vi "Main.vi"(11 "Module Admin":refnum<class "Delacor_lib_QMH_Cloneable Module Admin.lvclass">) -> ()   [LabVIEW 2020, in "FGen.lvlib"]
doc: "This template is based off of the Queued Message Handler design pattern and the Queued Message Handler project template that ships with LabVIEW.\n\nThe main difference is that the queue is private to this module and communication between modules is performed via Broadcast and Request events.\n\nRequest events are wrapped in public API methods and are handled in the Event Handling Loop (EHL) of this VI. Any module can register for Broadcast events sent by this module. The EHL generates messages based on user interface actions.\n\nThe Message Handling Loop (MHL) processes messages generated by the EHL, or by other messages. The messages are string values, so new messages can be added easily to the Message Cases case structure in the MHL. Each message cluster can also provide an optional value for Message Data, which is a variant that can be converted to whatever message-specific data is required.\n_____\nBased on DQMH Project Template 6.0.0.91."
uses:
  FGen.lvlib
  <vilib>/Delacor/Delacor QMH/Libraries/Message Queue_class/Delacor_lib_QMH_Message Queue.lvclass
  Module Data--cluster.ctl
  <vilib>/Utility/miscctls.llb/LVPointTypeDef.ctl
  <vilib>/Utility/error.llb/Error Cluster From Error Code.vi
  <vilib>/ErrorRing/Error Ring.xnode
  <vilib>/Delacor/Delacor QMH/Libraries/Message Queue_class/Delacor_lib_QMH_Enqueue Message (Single).vi
  Stop Argument--cluster.ctl
  <vilib>/Delacor/Delacor QMH/Libraries/Cloneable Module Admin_class/Delacor_lib_QMH_Cloneable Module Admin.lvclass
  Set Signal Type Argument--cluster.ctl
  Clases/Generador/Generador.lvclass
  Set to Default Argument--cluster.ctl
  Generate Signal (Reply Payload)--cluster.ctl
  Generate Signal Argument--cluster.ctl
  Oscilloscope Lista Argument--cluster.ctl
panel:
  out "error out":errorcluster
  out "Status":string
  in  "Simulate EHL Error":bool
  in  "Simulate MHL Error":bool
  # "Other QMH Modules communicate with this Module via its Public API (wrappers for its Request Events).\n\nThis Module communicates with other Modules via its Broadcast Events.\nAny module that wants to get these messages, just registers for this module's Broadcast events."
  # "This template is for the Delacor Modified Queued Message Handler design pattern.\n\nSee the block diagram for more information on how to use this template."
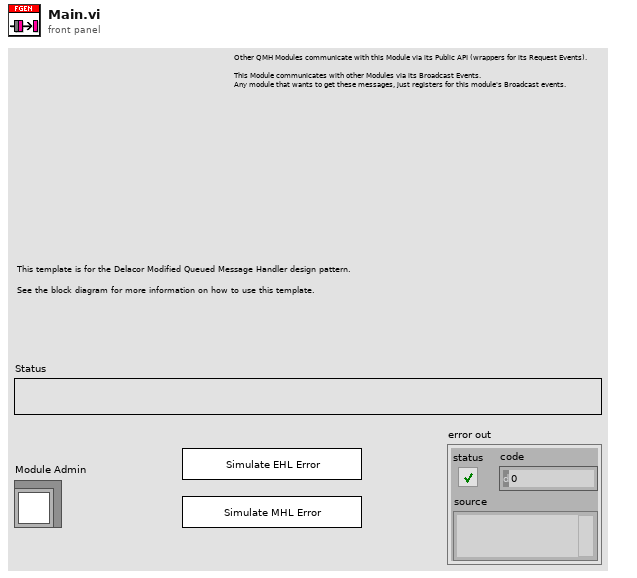
[diagram p1: front panel]
types:
  T1 = typedef "FGen.lvlib/Request Events--cluster.ctl" = cluster{"Stop Module":refnum<user-event>, "Show Panel":refnum<user-event>, "Hide Panel":refnum<user-event>, "Show Diagram":refnum<user-event>, "Get Module Execution Status":refnum<user-event>, "Set Signal Type":refnum<user-event>, "Set to Default":refnum<user-event>, "Generate Signal":refnum<user-event>}
  T2 = typedef "FGen.lvlib/Module Data--cluster.ctl" = cluster{"Status":string, "Generator":refnum<class "Generador.lvclass">}
  T3 = enum32{"invalid lock state", "Not Locked", "Locked (No Password)", "Password-protected"}
  T4 = typedef "FGen.lvlib/Stop Argument--cluster.ctl" = cluster{"Module ID":i32, "Origin":string, "Exit via Stop Module Req?":bool, "Wait for Module to stop?":bool}
  T5 = typedef "FGen.lvlib/Set Signal Type Argument--cluster.ctl" = cluster{"Module ID":i32, "signal type":enum16{"Sine Wave", "Triangle Wave", "Square Wave", "Sawtooth Wave"}}
  T6 = typedef "FGen.lvlib/Set to Default Argument--cluster.ctl" = cluster{"Module ID":i32, "Boolean":bool}
  T7 = typedef "FGen.lvlib/Generate Signal Argument--cluster.ctl" = cluster{"Module ID":i32, "Wait Notifier":refnum<notifier>, "wait for reply":bool}
  T8 = typedef "LVPointTypeDef.ctl" = cluster{"Horizontal":i16, "Vertical":i16}
  T9 = enum32{"Invalid", "Standard", "Closed", "Hidden", "Minimized", "Maximized"}
  T10 = typedef "FGen.lvlib/Generate Signal (Reply Payload)--cluster.ctl" = cluster{"signal out":waveform(dbl), "Generate Signal_error":errorcluster}
  T11 = typedef "FGen.lvlib/Oscilloscope Lista Argument--cluster.ctl" = cluster{"Module ID":i32, "Oscilloscopes Types":string[]}
  T12 = enum16{"Sine Wave", "Triangle Wave", "Square Wave", "Sawtooth Wave"}
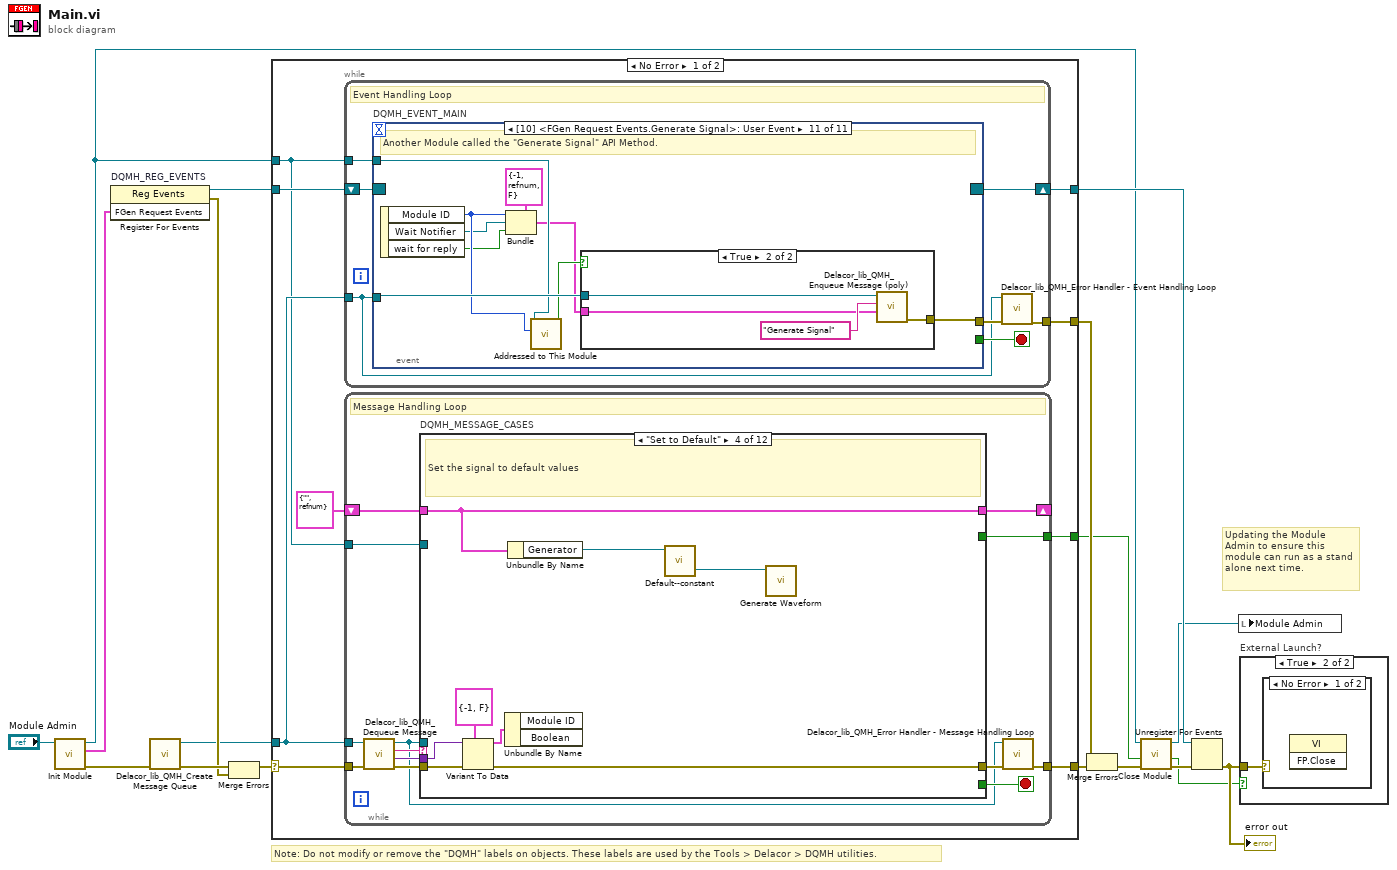
[diagram p0: block diagram]
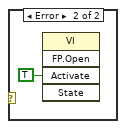
[diagram p3: hidden frame]
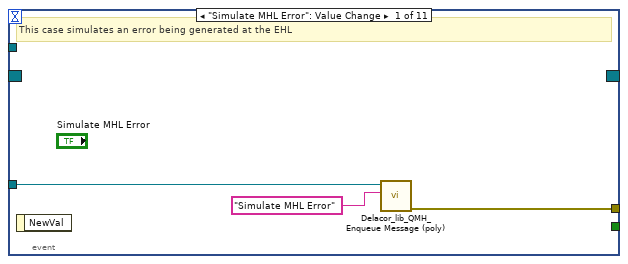
[diagram p4: hidden frame]
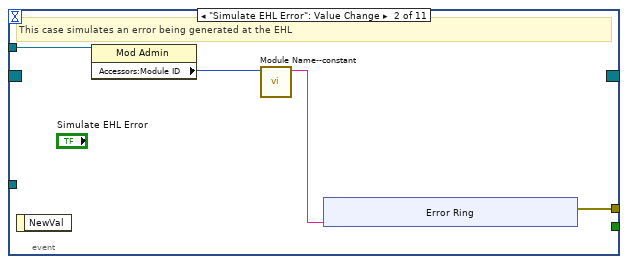
[diagram p5: hidden frame]
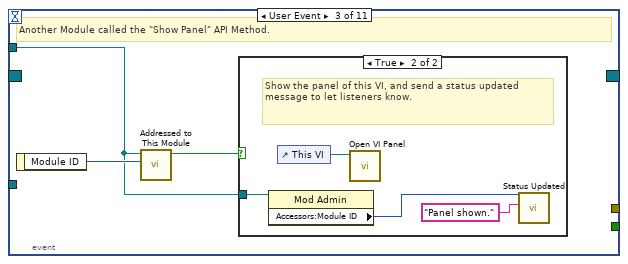
[diagram p6: hidden frame]
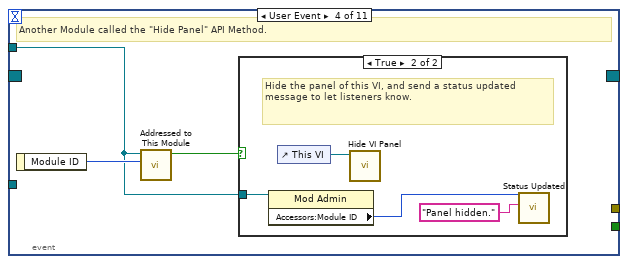
[diagram p8: hidden frame]
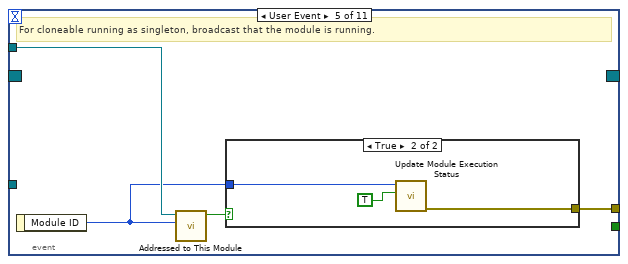
[diagram p10: hidden frame]
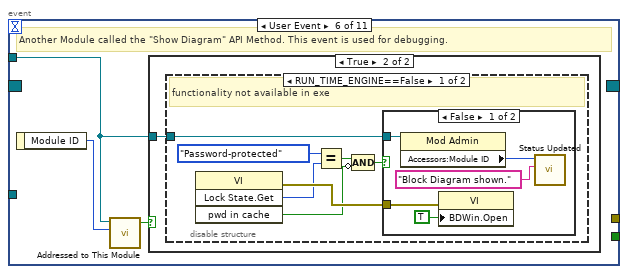
[diagram p12: hidden frame]
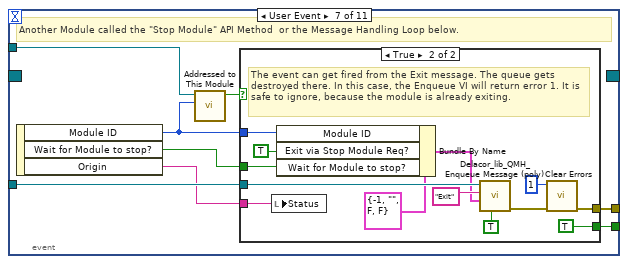
[diagram p16: hidden frame]
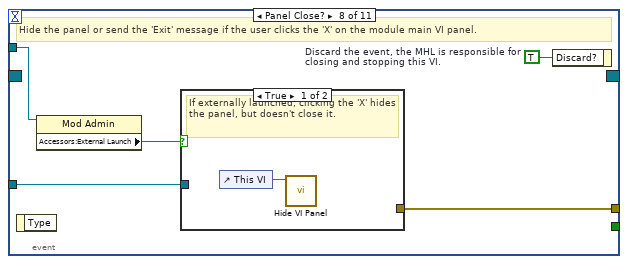
[diagram p18: hidden frame]
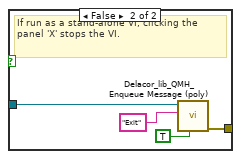
[diagram p19: hidden frame]
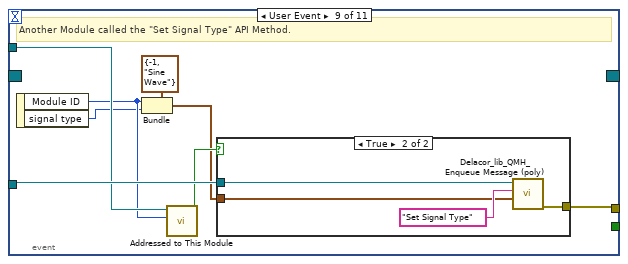
[diagram p20: hidden frame]
diagram:
  # "Note: Do not modify or remove the \"DQMH\" labels on objects. These labels are used by the Tools > Delacor > DQMH utilities."
  # "Updating the Module Admin to ensure this module can run as a stand alone next time."
  n1 = call "Init Module.vi"("Cloneable Module Admin in"="Module Admin") -> ("error out"=w15:errorcluster, "FGen Request Events"=w7:T1, "Cloneable Module Admin out"=w4:refnum<class "Delacor_lib_QMH_Cloneable Module Admin.lvclass">)  [unwired: 8 in]
  n2 = register-events "DQMH_REG_EVENTS"(w7) -> (reference out=w8:refnum<event-registration>, error out=w10:errorcluster)  [unwired: 2 in]
  n3 = call <vilib>:"Delacor_lib_QMH_Create Message Queue.vi"("error in"=w15) -> ("error out"=w12:errorcluster, "Message Queue"=w6:refnum<class "Delacor_lib_QMH_Message Queue.lvclass">)  [unwired: 9 in]
  n4 = Merge Errors(w12, w10) -> (w11:errorcluster)
  n5 = case shown="No Error" w11 {
    selector: w11 -> [w25 w300]
    tunnel: [w27 w299] -> w16
    tunnel: [w24 w307] -> w9
    tunnel: w8 -> [w22 w307]
    tunnel: w6 -> [w21 w298]
    tunnel: [w26 _] -> w17
    tunnel: w4 -> [w20 w303]
    tunnel: [w19 _] -> w2
    frame No Error {
      n6 = while {
        tunnel: w21 -> [w28]
        shift-right: [w31] -> w24
        shift-left: w22 -> [w32]
        tunnel: [w33] -> w26
        tunnel: w20 -> [w29]
        stop <- w30 stop-if-true
        # "Event Handling Loop"
        n7 = event "DQMH_EVENT_MAIN" shown="[10] <FGen Request Events.Generate Signal>: User Event" {
          selector: w32 -> [_ _ _ _ _ _ _ _ _ _ _]
          dyn-events: [_ _ _ _ _ _ _ _ _ _ _] -> w31
          timeout: _ -> [_ _ _ _ _ _ _ _ _ _ _]
          tunnel: [_ _ _ _ _ _ w89 _ _ _ _] -> w30
          tunnel: w28 -> [w36 _ _ _ _ _ w92 w108 w124 w136 w149]
          tunnel: [w37 w41 _ _ w66 _ w93 w111 w117 w129 w141] -> w34
          tunnel: w29 -> [_ w40 w49 w56 w64 w70 w91 w109 w122 w134 w147]
          event "Simulate MHL Error": Value Change {
            # "This case simulates an error being generated at the EHL"
            n8 = event-data() -> ()  [unwired: 1 in, 1 out]
            n9 = call-poly <vilib>:"Delacor_lib_QMH_Enqueue Message (poly).vi"("Message"="Simulate MHL Error", "Message Queue in"=w36) -> ("error out"=w37:errorcluster)  [unwired: 8 in, 1 out]
          }
          event "Simulate EHL Error": Value Change {
            # "This case simulates an error being generated at the EHL"
            n10 = event-data() -> ()  [unwired: 1 in, 1 out]
            n11 = property class="Mod Admin"(reference=w40) -> ("Accessors:Module ID"=w39:i32)  [unwired: 1 in, 2 out]
            n12 = call "Module Name--constant.vi"("Module ID"=w39) -> ("Module Name"=w38:string)  [unwired: 10 in]
            n13 = xnode "Error Ring"("parameter 0"=w38) -> ("error out"=w41:errorcluster)
          }
          event User Event {
            # "Another Module called the \"Show Panel\" API Method."
            n14 = event-data() -> ("Module ID"=w50:i32)  [unwired: 1 in]
            n15 = call "Addressed to This Module.vi"("Module ID from Argument"=w50, "Module Admin"=w49) -> ("Addressed to this instance?"=w51:bool)  [unwired: 8 in, 1 out]
            n16 = case shown="True" w51 {
              tunnel: w49 -> [_ w53]
              frame False {
              }
              frame True {
                # "Show the panel of this VI, and send a status updated message to let listeners know."
                n17 = property class="Mod Admin"(reference=w53) -> ("Accessors:Module ID"=w52:i32)  [unwired: 1 in, 2 out]
                n18 = control-ref of="This VI"() -> (w55:refnum<vi>)
                n19 = call "Open VI Panel.vi"("VI"=w55) -> ()  [unwired: 10 in, 1 out]
                n20 = call "Status Updated.vi"("Status"="Panel shown." ("format string"), "Module ID"=w52) -> ()  [unwired: 9 in, 1 out]
              }
            }
          }
          event User Event {
            # "Another Module called the \"Hide Panel\" API Method."
            n21 = event-data() -> ("Module ID"=w57:i32)  [unwired: 1 in]
            n22 = call "Addressed to This Module.vi"("Module ID from Argument"=w57, "Module Admin"=w56) -> ("Addressed to this instance?"=w58:bool)  [unwired: 8 in, 1 out]
            n23 = case shown="True" w58 {
              tunnel: w56 -> [_ w60]
              frame False {
              }
              frame True {
                # "Hide the panel of this VI, and send a status updated message to let listeners know."
                n24 = property class="Mod Admin"(reference=w60) -> ("Accessors:Module ID"=w59:i32)  [unwired: 1 in, 2 out]
                n25 = control-ref of="This VI"() -> (w62:refnum<vi>)
                n26 = call "Hide VI Panel.vi"("VI"=w62) -> ()  [unwired: 10 in, 1 out]
                n27 = call "Status Updated.vi"("Status"="Panel hidden." ("format string"), "Module ID"=w59) -> ()  [unwired: 9 in, 1 out]
              }
            }
          }
          event User Event {
            # "For cloneable running as singleton, broadcast that the module is running."
            n28 = event-data() -> ("Module ID"=w63:i32)  [unwired: 1 in]
            n29 = call "Addressed to This Module.vi"("Module ID from Argument"=w63, "Module Admin"=w64) -> ("Addressed to this instance?"=w65:bool)  [unwired: 8 in, 1 out]
            n30 = case shown="True" w65 {
              tunnel: [_ w69] -> w66
              tunnel: w63 -> [_ w68]
              frame False {
              }
              frame True {
                n31 = call "Update Module Execution Status.vi"("Running?"=TRUE, "Module ID"=w68) -> ("error out"=w69:errorcluster)  [unwired: 9 in]
              }
            }
          }
          event User Event {
            # "Another Module called the \"Show Diagram\" API Method. This event is used for debugging."
            n32 = event-data() -> ("Module ID"=w71:i32)  [unwired: 1 in]
            n33 = call "Addressed to This Module.vi"("Module ID from Argument"=w71, "Module Admin"=w70) -> ("Addressed to this instance?"=w72:bool)  [unwired: 8 in, 1 out]
            n34 = case shown="True" w72 {
              tunnel: w70 -> [_ w73]
              frame False {
              }
              frame True {
                n35 = disable-structure shown="RUN_TIME_ENGINE==False" {
                  disable-tunnel: w73 -> [w74 _]
                  frame condition #0 (active) {
                    # "functionality not available in exe"
                    n36 = invoke class="VI" method="Lock State.Get"() -> (error out=w80:errorcluster, "Get Lock State"=w79:T3, "pwd in cache"=w76:bool)  [unwired: 4 in, 1 out]
                    n37 = Equal?(x=T3."Password-protected", y=w79) -> (x = y?=w77:bool)
                    n38 = Compound Arithmetic op=AND(w77, invert w76) -> (w75:bool)
                    n39 = case shown="False" w75 {
                      tunnel: w80 -> [w85 _]
                      tunnel: w74 -> [w82 _]
                      frame False {
                        n40 = property class="Mod Admin"(reference=w82) -> ("Accessors:Module ID"=w81:i32)  [unwired: 1 in, 2 out]
                        n41 = property class="VI"(error in=w85, "BDWin.Open"=TRUE ("Block Diagram Window:Open")) -> ()  [unwired: 1 in, 2 out]
                        n42 = call "Status Updated.vi"("Status"="Block Diagram shown." ("format string"), "Module ID"=w81) -> ()  [unwired: 9 in, 1 out]
                      }
                      frame True {
                        # "Password-protected VI, and the password is not in the cache. Do not show the diagram."
                      }
                    }
                  }
                  frame condition #1 {
                  }
                }
              }
            }
          }
          event User Event {
            # "Another Module called the \"Stop Module\" API Method  or the Message Handling Loop below."
            n43 = event-data() -> ("Module ID"=w87:i32, "Wait for Module to stop?"=w88:bool, "Origin"=w86:string)  [unwired: 1 in]
            n44 = call "Addressed to This Module.vi"("Module ID from Argument"=w87, "Module Admin"=w91) -> ("Addressed to this instance?"=w90:bool)  [unwired: 8 in, 1 out]
            n45 = case shown="True" w90 {
              tunnel: [_ w105] -> w93
              tunnel: w92 -> [_ w101]
              tunnel: [_ TRUE] -> w89
              tunnel: w88 -> [_ w96]
              tunnel: w87 -> [_ w98]
              tunnel: w86 -> [_ w94]
              frame False {
              }
              frame True {
                # "The event can get fired from the Exit message. The queue gets destroyed there. In this case, the Enqueue VI will return error 1. It is safe to ignore, because the module is already exiting."
                n46 = local write "Status"(w94) -> ()
                n47 = Bundle By Name(cluster=T4 {"Module ID"=-1, "Origin"="", "Exit via Stop Module Req?"=FALSE, "Wait for Module to stop?"=FALSE} ("Stop Argument"), "Module ID"=w98, "Exit via Stop Module Req?"=TRUE, "Wait for Module to stop?"=w96) -> (w95:T4)
                n48 = call-poly <vilib>:"Delacor_lib_QMH_Enqueue Message (poly).vi"("Priority Message? (F)"=TRUE, "Message Data"=w95, "Message"="Exit", "Message Queue in"=w101) -> ("error out"=w106:errorcluster)  [unwired: 6 in, 1 out]
                n49 = call <vilib>:"Clear Errors.vi"("error in (no error)"=w106, "specific error code to clear (0: all)"=1) -> ("error out"=w105:errorcluster)  [unwired: 4 in, 1 out]
              }
            }
          }
          event Panel Close? {
            w110 = TRUE  # Discard the event, the MHL is responsible for closing and stopping this VI.
            # "Hide the panel or send the 'Exit' message if the user clicks the 'X' on the module main VI panel."
            n50 = event-data() -> ()  [unwired: 1 in, 1 out]
            n51 = property class="Mod Admin"(reference=w109) -> ("Accessors:External Launch"=w107:bool)  [unwired: 1 in, 2 out]
            n52 = case shown="True" w107 {
              tunnel: w108 -> [_ w115]
              tunnel: [_ w116] -> w111
              frame True {
                # "If externally launched, clicking the 'X' hides the panel, but doesn't close it."
                n53 = control-ref of="This VI"() -> (w112:refnum<vi>)
                n54 = call "Hide VI Panel.vi"("VI"=w112) -> ()  [unwired: 10 in, 1 out]
              }
              frame False {
                # "If run as a stand-alone VI, clicking the panel 'X' stops the VI."
                n55 = call-poly <vilib>:"Delacor_lib_QMH_Enqueue Message (poly).vi"("Priority Message? (F)"=TRUE, "Message"="Exit", "Message Queue in"=w115) -> ("error out"=w116:errorcluster)  [unwired: 7 in, 1 out]
              }
            }
            n56 = event-data("Discard?"=w110) -> ()  [unwired: 1 in, 1 out]
          }
          event User Event {
            # "Another Module called the \"Set Signal Type\" API Method."
            n57 = event-data() -> ("Module ID"=w119:i32, "signal type"=w118:T12)  [unwired: 1 in]
            n58 = Bundle(cluster=T5 {"Module ID"=-1, "signal type"=enum."Sine Wave"} ("Set Signal Type Argument"), "Module ID"=w119, "signal type"=w118) -> (w120:T5)
            n59 = call "Addressed to This Module.vi"("Module ID from Argument"=w119, "Module Admin"=w122) -> ("Addressed to this instance?"=w123:bool)  [unwired: 8 in, 1 out]
            n60 = case shown="True" w123 {
              tunnel: w124 -> [_ w128]
              tunnel: w120 -> [_ w126]
              tunnel: [_ w125] -> w117
              frame False {
              }
              frame True {
                n61 = call-poly <vilib>:"Delacor_lib_QMH_Enqueue Message (poly).vi"("Message Data"=w126, "Message"="Set Signal Type", "Message Queue in"=w128) -> ("error out"=w125:errorcluster)  [unwired: 7 in, 1 out]
              }
            }
          }
          event User Event {
            # "Another Module called the \"Set to Default\" API Method."
            n62 = event-data() -> ("Module ID"=w131:i32, "Boolean"=w130:bool)  [unwired: 1 in]
            n63 = Bundle(cluster=T6 {"Module ID"=-1, "Boolean"=FALSE} ("Set to Default Argument"), "Module ID"=w131, "Boolean"=w130) -> (w132:T6)
            n64 = call "Addressed to This Module.vi"("Module ID from Argument"=w131, "Module Admin"=w134) -> ("Addressed to this instance?"=w135:bool)  [unwired: 8 in, 1 out]
            n65 = case shown="True" w135 {
              tunnel: w136 -> [_ w140]
              tunnel: w132 -> [_ w138]
              tunnel: [_ w137] -> w129
              frame False {
              }
              frame True {
                n66 = call-poly <vilib>:"Delacor_lib_QMH_Enqueue Message (poly).vi"("Message Data"=w138, "Message"="Set to Default", "Message Queue in"=w140) -> ("error out"=w137:errorcluster)  [unwired: 7 in, 1 out]
              }
            }
          }
          event User Event {
            # "Another Module called the \"Generate Signal\" API Method."
            n67 = event-data() -> ("Module ID"=w144:i32, "Wait Notifier"=w143:refnum<notifier>, "wait for reply"=w142:bool)  [unwired: 1 in]
            n68 = Bundle(cluster=T7 {"Module ID"=-1, "Wait Notifier"=refnum, "wait for reply"=FALSE} ("Generate Signal Argument"), "Module ID"=w144, "Wait Notifier"=w143, "wait for reply"=w142) -> (w145:T7)
            n69 = call "Addressed to This Module.vi"("Module ID from Argument"=w144, "Module Admin"=w147) -> ("Addressed to this instance?"=w148:bool)  [unwired: 8 in, 1 out]
            n70 = case shown="True" w148 {
              tunnel: w149 -> [_ w153]
              tunnel: w145 -> [_ w151]
              tunnel: [_ w150] -> w141
              frame False {
              }
              frame True {
                n71 = call-poly <vilib>:"Delacor_lib_QMH_Enqueue Message (poly).vi"("Message Data"=w151, "Message"="Generate Signal", "Message Queue in"=w153) -> ("error out"=w150:errorcluster)  [unwired: 7 in, 1 out]
              }
            }
          }
        }
        n72 = call-dynamic "Delacor_lib_QMH_Error Handler - Event Handling Loop.vi"("error in"=w34, "Message Queue in"=w28) -> ("dup error in"=w33:errorcluster)  [unwired: 8 in, 1 out]
      }
      n73 = while {
        tunnel: w21 -> [w157]
        shift-right: [w161] -> _
        shift-left: T2 {"Status"="", "Generator"=refnum} ("Data Cluster") -> [w162]
        tunnel: w25 -> [w165]
        tunnel: [w163] -> w27
        tunnel: w20 -> [w155]
        tunnel: [w154] -> w19
        stop <- w160 stop-if-true
        # "Message Handling Loop"
        n74 = call-dynamic "Delacor_lib_QMH_Dequeue Message.vi"("error in"=w165, "Message Queue in"=w157) -> ("error out"=w164:errorcluster, "Message Data"=w158:variant, "Message"=w159:string, "Message Queue out"=w156:refnum<class "Delacor_lib_QMH_Message Queue.lvclass">)  [unwired: 6 in]
        n75 = case "DQMH_MESSAGE_CASES" shown="\"Set to Default\"" w159 {
          selector: w159 -> [_ _ _ _ _ _ _ _ _ _ _ w285]
          tunnel: w156 -> [_ _ _ _ _ _ _ _ w236 _ w275 _]
          tunnel: w164 -> [w186 w190 w198 w206 w221 w229 w232 w234 w245 w258 w281 w287]
          tunnel: [w184 w190 w197 w205 w211 w227 w231 w234 w241 w257 w278 w288] -> w166
          tunnel: w162 -> [w177 w189 w193 w201 w220 w228 w230 w233 w240 w255 w274 w286]
          tunnel: [w176 w189 w193 w201 w220 w228 w230 w233 w240 w255 w274 w286] -> w161
          tunnel: [_ _ _ _ _ _ _ _ _ _ w273 _] -> w160
          tunnel: w158 -> [_ _ w196 w204 w218 w226 _ _ w239 _ w271 _]
          tunnel: w155 -> [w172 _ _ _ _ _ _ _ w238 w253 w267 w283]
          tunnel: [_ _ _ _ _ _ _ _ _ _ w269 _] -> w154
          frame "Initialize" {
            w169 = "Initial Message" ("Initial Message")
            # "Initialize - Any operation that needs to be done before the module can receive messages. Synchronize Caller Events.vi will inform Start Module.vi that the module has launched and is ready to receive messages. Module Did Init.vi will broadcast that the module initialized."
            n76 = call "Synchronize Caller Events.vi"("error in (no error)"=w186, "Module Admin"=w172) -> ("error out"=w185:errorcluster, "Module Admin out"=w171:refnum<class "Delacor_lib_QMH_Cloneable Module Admin.lvclass">)  [unwired: 8 in]
            n77 = property class="Mod Admin"(reference=w171) -> ("Accessors:Module ID"=w168:i32, "Accessors:External Launch"=w173:bool)  [unwired: 1 in, 2 out]
            n78 = call "Get Classes Names.vi"() -> ("Classes"=w167:string[])  [unwired: 11 in]
            n79 = call "Module Name--constant.vi"("Module ID"=w168) -> ("Module Name"=w181:string)  [unwired: 10 in]
            n80 = call "Oscilloscope Lista.vi"("Oscilloscopes Types"=w167, "Module ID"=w168) -> ()  [unwired: 9 in, 1 out]
            n81 = property class="VI"("Front Panel.Title"=w181) -> (reference out=w183:refnum<vi>, error out=w188:errorcluster)  [unwired: 2 in]
            n82 = Select(t=T9."Hidden" ("State"), s=w173, f=T9."Standard" ("State")) -> (s? t:f=w178:T9)
            n83 = invoke class="VI" method="FP.Open"(reference=w183, error in=w188, "State"=w178) -> (reference out=w182:refnum<vi>, error out=w187:errorcluster)  [unwired: 2 in, 3 out]
            n84 = call "Module Name--constant.vi"("Module ID"=w168) -> ("Module Name"=w174:string)  [unwired: 10 in]
            n85 = Bundle By Name(cluster=w177, "Status"=w169) -> (w176:T2)
            n86 = invoke class="VI" method="FP.Center"(reference=w182, error in=w187) -> ()  [unwired: 1 in, 3 out]
            n87 = property on="Pane" class="Pane"("Origin"=T8 {"Horizontal"=0, "Vertical"=0}) -> ()  [unwired: 2 in, 2 out]
            n88 = call "Module Did Init.vi"("error in (no error)"=w185, "Initialized?"=TRUE, "Origin"=w174, "Module ID"=w168) -> ("error out"=w184:errorcluster)  [unwired: 7 in]
            "Status" <- w169
          }
          frame "---Module Specific---" {
            # "Separator -- The following cases handle messages specific to this Module."
          }
          frame "Set Signal Type" {
            # "#CompleteMissingCode\nAdd the output Object of the method to the Module Data"
            # "Set the Signal type to be generated"
            n89 = Variant To Data(error in=w198, type=T5 {"Module ID"=-1, "signal type"=enum."Sine Wave"} ("Set Signal Type Argument"), Variant=w196) -> (data=w194:T5, error out=w197:errorcluster)
            n90 = Unbundle By Name(w194) -> ("signal type"=w191:T12)
            n91 = Unbundle By Name(w193) -> ("Generator"=w192:refnum<class "Generador.lvclass">)
            n92 = call "Set signal type.vi"("signal type"=w191, "Generator in"=w192) -> ()  [unwired: 8 in, 2 out]
          }
          frame "Set to Default" {
            # "Set the signal to default values"
            n93 = Variant To Data(error in=w206, type=T6 {"Module ID"=-1, "Boolean"=FALSE} ("Set to Default Argument"), Variant=w204) -> (data=w202:T6, error out=w205:errorcluster)
            n94 = Unbundle By Name(w202) -> ()  [unwired: 2 out]
            n95 = Unbundle By Name(w201) -> ("Generator"=w200:refnum<class "Generador.lvclass">)
            n96 = call-dynamic "Default--constant.vi"("Generator in"=w200) -> ("Generator out"=w199:refnum<class "Generador.lvclass">)  [unwired: 9 in, 1 out]
            n97 = call "Generate Waveform.vi"("Generator in"=w199) -> ()  [unwired: 8 in, 3 out]
          }
          frame "Generate Signal" {
            # "Generate the signal with the Defined values"
            n98 = Variant To Data(error in=w221, type=T7 {"Module ID"=-1, "Wait Notifier"=refnum, "wait for reply"=FALSE} ("Generate Signal Argument"), Variant=w218) -> (data=w216:T7, error out=w219:errorcluster)
            n99 = Unbundle By Name(w216) -> ("Wait Notifier"=w215:refnum<notifier>, "wait for reply"=w214:bool)
            n100 = call-dynamic "Default--constant.vi"("Generator in"=refnum<class "Generador.lvclass"> refnum ("FGen.lvlib:Generator")) -> ("Generator out"=w208:refnum<class "Generador.lvclass">)  [unwired: 9 in, 1 out]
            n101 = call "Generate Waveform.vi"("Generator in"=w208) -> ("error out"=w207:errorcluster, "Waveform"=w210:waveform(dbl))  [unwired: 8 in, 1 out]
            n102 = Bundle By Name(cluster=T10 {"signal out"={"t0"=timestamp(0 s since 1904-01-01), "dt"=1.0, "Y"=[]}, "Generate Signal_error"={"status"=FALSE, "code"=0, "source"=""}} ("Generate Signal (Reply Payload)"), "signal out"=w210) -> (w213:T10)  [unwired: 1 in]
            n103 = case shown="True" w214 {
              tunnel: w215 -> [_ w223]
              tunnel: w213 -> [_ w222]
              frame False {
              }
              frame True {
                n104 = Send Notification(notification=w222, notifier=w223) -> ()  [unwired: 1 in, 2 out]
              }
            }
            n105 = Merge Errors(w219, w207) -> (w211:errorcluster)
          }
          frame "Oscilloscope List" {
            # "#Code_Review_Todo The DQMH event associated with this message case has been removed. Consider removing this frame if this message is no longer needed. Delete this label if this code is still required."
            # "#CodeNeeded\n1. Configure this Message Case for handling the \"Oscilloscope List\" message.\n2. Delete or edit this label when done."
            n106 = Variant To Data(error in=w229, type=T11 {"Module ID"=-1, "Oscilloscopes Types"=[]} ("Oscilloscope List Argument"), Variant=w226) -> (data=w224:T11, error out=w227:errorcluster)
            n107 = Unbundle By Name(w224) -> ()  [unwired: 2 out]
          }
          frame "---Copy This Frame---" {
            # "Duplicate this frame when creating new messages.  Change this comment in the duplicated frame to describe this message."
            n108 = Merge Errors(w232) -> (w231:errorcluster)
          }
          frame "---Exit and Error Handling---" {
            # "Separator - the following cases handle errors and exit messages."
          }
          frame "Error" {
            # "Error - Check the error message data and respond accordingly. This message is sent by the \"Error Handler\" VIs at the end of each loop in this application."
            n109 = property class="Mod Admin"(reference=w238) -> ("Accessors:External Launch"=w237:bool, "Accessors:Module ID"=w235:i32)  [unwired: 1 in, 2 out]
            n110 = Variant To Data(error in=w245, type=errorcluster {"status"=FALSE, "code"=0, "source"=""} ("error constant"), Variant=w239) -> (data=w246:errorcluster, error out=w243:errorcluster)
            n111 = call "Error Reported.vi"("Error"=w246, "Module ID"=w235) -> ()  [unwired: 9 in, 1 out]
            n112 = case shown="False" w237 {
              tunnel: [w251 _] -> w242
              tunnel: w236 -> [w249 _]
              tunnel: w246 -> [w250 _]
              frame False {
                # "If the module is running standalone, then pop up an error dialog and call the \"Exit\" message."
                n113 = call <vilib>:"Simple Error Handler.vi"("error in (no error)"=w250) -> ()  [unwired: 4 in, 5 out]
                n114 = call-poly <vilib>:"Delacor_lib_QMH_Enqueue Message (poly).vi"("Priority Message? (F)"=TRUE, "Message"="Exit", "Message Queue in"=w249) -> ("error out"=w251:errorcluster)  [unwired: 7 in, 1 out]
              }
              frame True {
                # "If the module was launched externally, calling the Error Reported broadcast VI is the only action performed by the \"Error\" message. The module's caller can then process the error appropriately."
              }
            }
            n115 = Merge Errors(w243, w242) -> (w241:errorcluster)
            n116 = local write "error out"(w241) -> ()
          }
          frame "Simulate MHL Error" {
            # "Simulate an error occurring at the MHL"
            n117 = property class="Mod Admin"(reference=w253) -> ("Accessors:Module ID"=w254:i32)  [unwired: 1 in, 2 out]
            n118 = call "Module Name--constant.vi"("Module ID"=w254) -> ("Module Name"=w252:string)  [unwired: 10 in]
            n119 = xnode "Error Ring"("parameter 0"=w252) -> ("error out"=w256:errorcluster)
            n120 = Merge Errors(w258, w256) -> (w257:errorcluster)
          }
          frame "Exit" {
            w272 = 91  # 91: not all Exit messages will have an argument
            w273 = TRUE  # Stop the VI
            # "Release the message queue reference"
            # "Exit - Exit the application."
            n121 = Variant To Data(error in=w281, type=T4 {"Module ID"=-1, "Origin"="", "Exit via Stop Module Req?"=FALSE, "Wait for Module to stop?"=FALSE} ("Stop Argument"), Variant=w271) -> (data=w268:T4, error out=w276:errorcluster)
            n122 = call <vilib>:"Clear Errors.vi"("error in (no error)"=w276, "specific error code to clear (0: all)"=w272) -> ("error out"=w280:errorcluster)  [unwired: 4 in, 1 out]
            n123 = control-ref of="This VI"() -> (w266:refnum<vi>)
            n124 = call-dynamic "Delacor_lib_QMH_Release Message Queue.vi"("error in"=w280, "Message Queue"=w275) -> ("error out"=w279:errorcluster)  [unwired: 9 in]
            n125 = call "Handle Exit.vi"("Stop Argument"=w268, "Module Admin in"=w267, "VI reference"=w266) -> ("error out"=w277:errorcluster, "Wait for Stop?"=w269:bool)  [unwired: 7 in]
            n126 = Merge Errors(w279, w277) -> (w278:errorcluster)
          }
          frame Default {
            # "'Default' case only runs if there is a message that isn't defined in any of the other cases.  Output a programming error."
            n127 = property class="Mod Admin"(reference=w283) -> ("Accessors:Module ID"=w282:i32)  [unwired: 1 in, 2 out]
            n128 = call "Module Name--constant.vi"("Module ID"=w282) -> ("Module Name"=w284:string)  [unwired: 10 in]
            n129 = xnode "Error Ring"("parameter 0"=w285, "parameter 1"=w284) -> ("error out"=w289:errorcluster)
            n130 = Merge Errors(w287, w289) -> (w288:errorcluster)
          }
        }
        n131 = call-dynamic "Delacor_lib_QMH_Error Handler - Message Handling Loop.vi"("error in"=w166, "Message Queue in"=w156) -> ("dup error in"=w163:errorcluster)  [unwired: 8 in, 1 out]
      }
    }
    frame Error {
      n132 = call "Synchronize Caller Events.vi"("Module Admin"=w303) -> ("Module Admin out"=w302:refnum<class "Delacor_lib_QMH_Cloneable Module Admin.lvclass">)  [unwired: 9 in, 1 out]
      n133 = property class="Mod Admin"(reference=w302) -> ("Accessors:Module ID"=w301:i32)  [unwired: 1 in, 2 out]
      n134 = call-dynamic "Delacor_lib_QMH_Release Message Queue.vi"("error in"=w300, "Message Queue"=w298) -> ("error out"=w299:errorcluster)  [unwired: 9 in]
      n135 = call "Module Name--constant.vi"("Module ID"=w301) -> ("Module Name"=w306:string)  [unwired: 10 in]
      n136 = Format Into String(format string="An error occurred during initialization. %s is no longer running.", w306) -> (resulting string=w304:string)  [unwired: 2 in, 1 out]
      n137 = call "Error Reported.vi"("Additional Information"=w304, "Error"=w299, "Module ID"=w301) -> ()  [unwired: 8 in, 1 out]
    }
  }
  n138 = Merge Errors(w17, w16) -> (w18:errorcluster)
  n139 = call "Close Module.vi"("error in"=w18, "Wait for stop?"=w2, "Module Admin in"=w4) -> ("error out"=w14:errorcluster, "External Launch"=w1:bool, "Module Admin out"=w3:refnum<class "Delacor_lib_QMH_Cloneable Module Admin.lvclass">)  [unwired: 6 in]
  n140 = Unregister For Events(event registration refnum=w9, error in=w14) -> (error out=w13:errorcluster)
  "error out" <- w13
  n141 = local write "Module Admin"(w3) -> ()
  n142 = case "External Launch?" shown="True" w1 {
    tunnel: w13 -> [_ w308]
    frame False {
    }
    frame True {
      n143 = case shown="No Error" w308 {
        frame No Error {
          n144 = invoke class="VI" method="FP.Close"() -> ()  [unwired: 3 in, 3 out]
        }
        frame Error {
          n145 = invoke class="VI" method="FP.Open"("Activate"=TRUE ("Activate?")) -> ()  [unwired: 4 in, 5 out]
        }
      }
    }
  }
